vi "Introduccion.vi"() -> ()   [LabVIEW 2015]
panel:
  in  "Num 2":dbl
  out "String 2":string
  in  "String":string
  out "Boolean 2":bool
  in  "Boolean":bool
  out "Time Stamp 2":timestamp
  in  "Time Stamp":timestamp
  out "Salida con variables":dbl
  in  "Num 1":dbl
  in  "Ingresa otro numero":dbl
  out "Resultado":dbl
  in  "Ingresa un numero":dbl
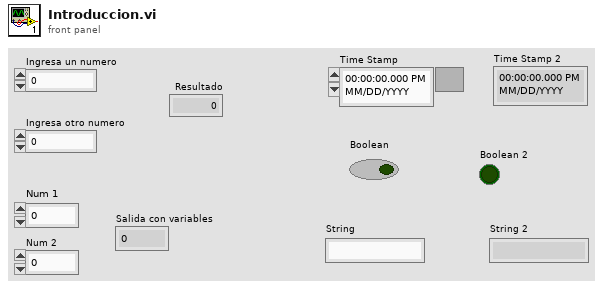
[diagram p1: front panel]
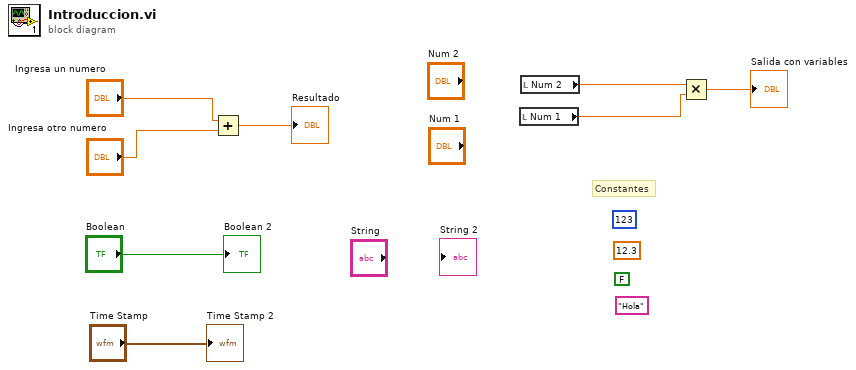
[diagram p0: block diagram]
diagram:
  (unwired) "Hola"
  (unwired) FALSE
  (unwired) 12.3
  (unwired) 123
  # "Constantes"
  n1 = Add(x="Ingresa un numero", y="Ingresa otro numero") -> (x+y=→"Resultado":dbl)
  n2 = local read "Num 1"() -> (w3:dbl)
  n3 = local read "Num 2"() -> (w4:dbl)
  n4 = Multiply(x=w4, y=w3) -> (x*y=→"Salida con variables":dbl)
  "Time Stamp 2" <- "Time Stamp"
  "Boolean 2" <- "Boolean"
